vi "c ctre phoenixpro deserialize pgn.vi"(6 "framePeriodMs":u16, 7 "frame_index":u16, 8 "error in (no error)":errorcluster, 9 "strlen":u32, 10 "str":string, 11 "spn":i32) -> (0 "error out":errorcluster, 3 "function return":i32, 4 "framePeriodMs out":u16, 5 "frame_index out":u16)   [LabVIEW 2020, in "CTRE_PhoenixTools.lvlib"]
doc: "CTREXPORT int c_ctre_phoenixpro_deserialize_pgn(int spn, const char *str, uint32_t strlen, uint16_t *frame_index, uint16_t *framePeriodMs);"
uses:
  <userlib>/CTRE_PhoenixTools/CTRE_PhoenixTools.lvlib
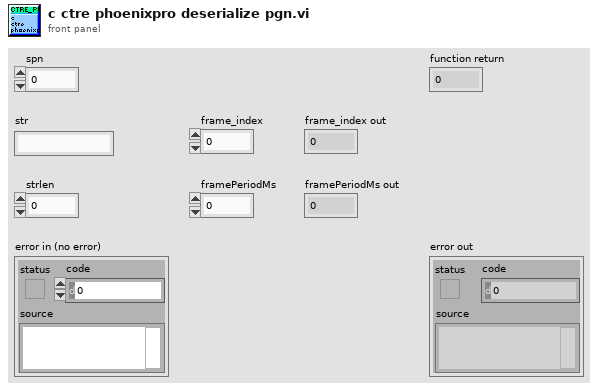
[diagram p1: front panel]
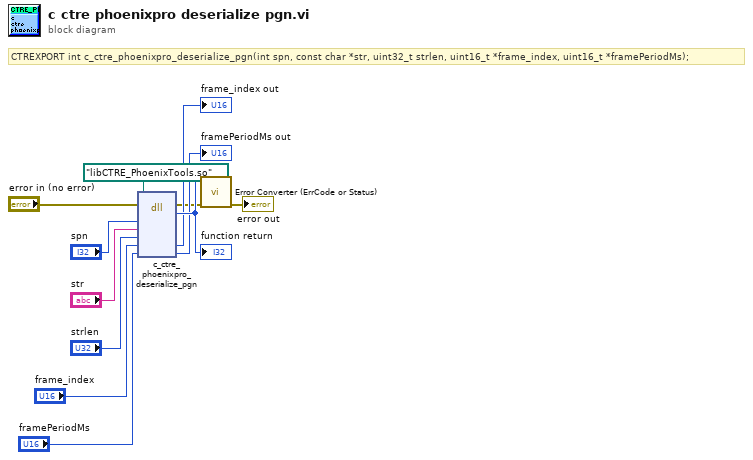
[diagram p0: block diagram]
diagram:
  # "CTREXPORT int c_ctre_phoenixpro_deserialize_pgn(int spn, const char *str, uint32_t strlen, uint16_t *frame_index, uint16_t *framePeriodMs);"
  n1 = dll-call lib="?" fn="c_ctre_phoenixpro_deserialize_pgn"(path in=path "libCTRE_PhoenixTools.so", error in="error in (no error)", "spn"="spn", "str"="str", "strlen"="strlen", "frame_index"="frame_index", "framePeriodMs"="framePeriodMs") -> (error out=w3:errorcluster, w12:i32, "frame_index"=→"frame_index out":u16, "framePeriodMs"=→"framePeriodMs out":u16)  [unwired: 4 in, 1 out]
  "function return" <- w12
  n2 = call <userlib>:"Error Converter (ErrCode or Status).vi"("error in (no error)"=w3, "error code"=w12) -> ("error out"=→"error out":errorcluster)  [unwired: 9 in]
